vi "HDF5_Write_Tone_Record.vi"(0 "ToneRef":T5 {"Downshift_dset" format="%.0x"; "DeltaPhase_dset" format="%.0x"; "Phase_dset" format="%.0x"; "SNR_dset" format="%.0x"; "df_dset" format="%.0x"; "PeakLoc_dset" format="%.0x"; "MaxValue_dset" format="%.0x"; "TImeStamp_dset" format="%.0x"; "TimeString_dset" format="%.0x"}, 5 "TargetToneData":T1={"Cal"={"Shift_"=-24999462.633451957, "Peak_ToFPGA"=-24999462.633451957, "MaxValue"=0.0, "MaxIndex"=0, "Tone"={"PkLocTrak"=0.0, "PkLocDisp"=0.0, "df_"=0.0, "ZoomPwr"=[], "Phase"=0.0, "PhaseOld"=0.0, "AboveThresh?"=FALSE, "MaxI"=0.0, "MaxQ"=0.0, "median"=0.0, "ISpect"=[], "QSpect"=[], "DeltaPhase"=0.0}, "TimeDomainI"=array[12500 elements], "TimeDomainQ"=[], "PwrSpectrum"=array[12500 elements], "RunningAvgFreq"=0.0, "ISpectPos"=[], "ISpectNeg"=[], "QSpectPos"=[], "QSpectNeg"=[], "10Hz_PwrSpectr"=[], "SNR"=0.0, "AliasWarn"=FALSE, "10Hz_Peak"=[], "ISpect+-"=[], "QSpect+-"=[], "TimeStamp"=timestamp(0 s since 1904-01-01), "I_Index"=array[12500 elements], "Q_Index"=array[12500 elements], "10MHz"=FALSE}, "Beac"={"Shift_"=-24999462.633451957, "Peak_ToFPGA"=-24999462.633451957, "MaxValue"=0.0, "MaxIndex"=0, "Tone"={"PkLocTrak"=0.0, "PkLocDisp"=0.0, "df_"=0.0, "ZoomPwr"=[], "Phase"=0.0, "PhaseOld"=0.0, "AboveThresh?"=FALSE, "MaxI"=0.0, "MaxQ"=0.0, "median"=0.0, "ISpect"=[], "QSpect"=[], "DeltaPhase"=0.0}, "TimeDomainI"=array[12500 elements], "TimeDomainQ"=[], "PwrSpectrum"=array[12500 elements], "RunningAvgFreq"=0.0, "ISpectPos"=[], "ISpectNeg"=[], "QSpectPos"=[], "QSpectNeg"=[], "10Hz_PwrSpectr"=[], "SNR"=0.0, "AliasWarn"=FALSE, "10Hz_Peak"=[], "ISpect+-"=[], "QSpect+-"=[], "TimeStamp"=timestamp(0 s since 1904-01-01), "I_Index"=array[12500 elements], "Q_Index"=array[12500 elements], "10MHz"=FALSE}, "Time"=[], "Saturat"={"MeasMean0"=0.0, "MeasMean1"=0.0, "MeasMax"=0.0, "1_Max"=0.0, "4_Max"=0.0, "5_Max"=0.0, "6_Max"=0.0, "7_Max"=0.0}} {"Beac"."Tone"."median" format="%0.2f"; "Beac"."Tone"."MaxQ" format="%0.2f"; "Cal"."Tone"."median" format="%0.2f"; "Cal"."Tone"."MaxQ" format="%0.2f"}, 11 "error in":errorcluster) -> (15 "error out":errorcluster)   [LabVIEW 2018]
doc: "Write a single Tone<x> record with timestamp:\nTone1\n Beac - cluster\n BeacZoom - 1024 element Double array (waveform) \n Cal - cluster\n CalZoom - 1024 element Double array (waveform)"
uses:
  <vilib>/addons/h5labview2/dataset/H5D.lvlib
  <vilib>/addons/h5labview2/base/H5Equery.vi
  lib_path_mod_20200519.vi
  <vilib>/addons/h5labview2/dataset/H5Dwrite.llb/H5Dwrite.xnode
  <vilib>/addons/h5labview2/space/H5S.lvlib
  <vilib>/addons/h5labview2/base/hid_t_renamed.ctl
  HDF5_Tone_refs.ctl
  Controls/ToneInfoClust.ctl
  Controls/Clusts/ChannelToneData.ctl
  Controls/Clusts/TargetToneData.ctl
  Controls/Clusts/SaturationMonitor.ctl
  <vilib>/addons/h5labview2/base/hid_t.ctl
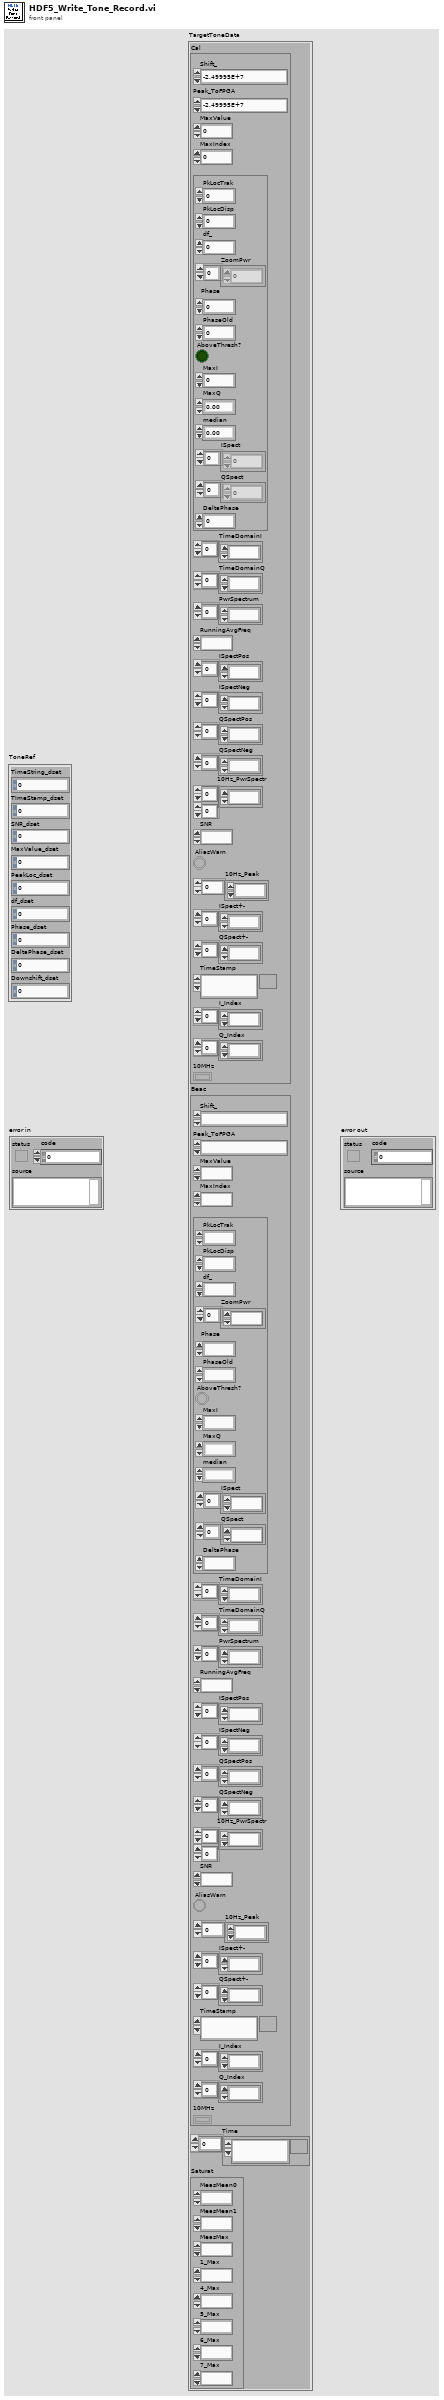
[diagram p1: front panel]
types:
  T1 = typedef "TargetToneData.ctl" = cluster{"Cal":T2, "Beac":T2, "Time":timestamp[], "Saturat":T4}
  T2 = typedef "ChannelToneData.ctl" = cluster{"Shift_":dbl, "Peak_ToFPGA":dbl, "MaxValue":dbl, "MaxIndex":i32, "Tone":T3, "TimeDomainI":ext[], "TimeDomainQ":ext[], "PwrSpectrum":dbl[], "RunningAvgFreq":dbl, "ISpectPos":dbl[], "ISpectNeg":dbl[], "QSpectPos":dbl[], "QSpectNeg":dbl[], "10Hz_PwrSpectr":dbl[][], "SNR":dbl, "AliasWarn":bool, "10Hz_Peak":dbl[], "ISpect+-":dbl[], "QSpect+-":dbl[], "TimeStamp":timestamp, "I_Index":ext[], "Q_Index":ext[], "10MHz":bool}
  T3 = typedef "ToneInfoClust.ctl" = cluster{"PkLocTrak":dbl, "PkLocDisp":dbl, "df_":dbl, "ZoomPwr":dbl[], "Phase":dbl, "PhaseOld":dbl, "AboveThresh?":bool, "MaxI":dbl, "MaxQ":dbl, "median":dbl, "ISpect":dbl[], "QSpect":dbl[], "DeltaPhase":dbl}
  T4 = typedef "SaturationMonitor.ctl" = cluster{"MeasMean0":dbl, "MeasMean1":dbl, "MeasMax":dbl, "1_Max":dbl, "4_Max":dbl, "5_Max":dbl, "6_Max":dbl, "7_Max":dbl}
  T5 = typedef "HDF5_Tone_refs.ctl" = cluster{"TimeString_dset":T6, "TImeStamp_dset":T6, "SNR_dset":T6, "MaxValue_dset":T6, "PeakLoc_dset":T6, "df_dset":T6, "Phase_dset":T6, "DeltaPhase_dset":T6, "Downshift_dset":T6}
  T6 = typedef "hid_t.ctl" = i32
  T7 = typedef "HDF5_ToneInfoClust.ctl" = cluster{"Timestring":string, "Timestamp":dbl, "MaxValue":dbl, "PeakLoc":dbl, "df":dbl}
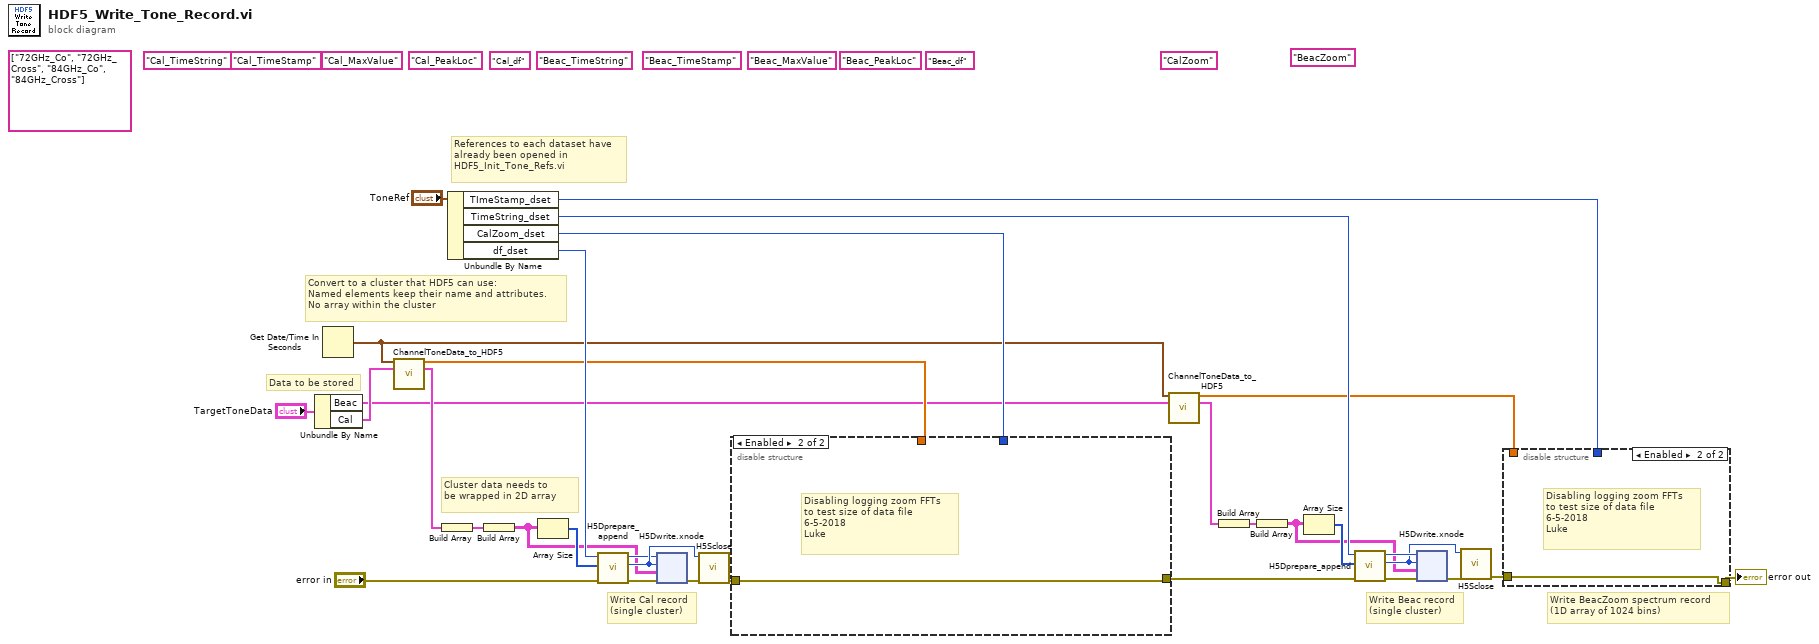
[diagram p0: block diagram]
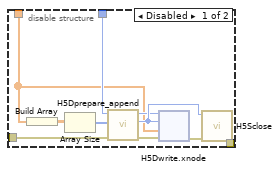
[diagram p2: hidden frame]
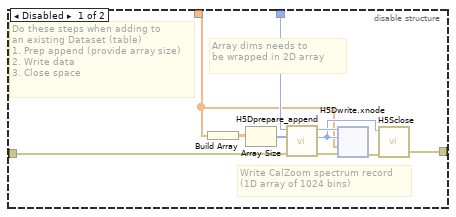
[diagram p3: hidden frame]
diagram:
  (unwired) "Beac_df" ("string")
  (unwired) "Beac_PeakLoc" ("string")
  (unwired) "Beac_MaxValue" ("string")
  w1 = "Beac_TimeStamp" ("string")
  w2 = "Beac_TimeString" ("string")
  (unwired) "Cal_df" ("string")
  (unwired) "Cal_PeakLoc" ("string")
  (unwired) "Cal_MaxValue" ("string")
  (unwired) "Cal_TimeStamp" ("string")
  (unwired) "BeacZoom" ("string")
  w3 = "CalZoom" ("string")
  (unwired) "Cal_TimeString" ("string")
  (unwired) string[] ["72GHz_Co", "72GHz_Cross", "84GHz_Co", "84GHz_Cross"]
  # "Convert to a cluster that HDF5 can use:\nNamed elements keep their name and attributes.\nNo array within the cluster"
  # "Cluster data needs to \nbe wrapped in 2D array"
  # "Data to be stored"
  # "References to each dataset have \nalready been opened in \nHDF5_Init_Tone_Refs.vi"
  # "Write BeacZoom spectrum record\n(1D array of 1024 bins)"
  # "Write Beac record\n(single cluster)"
  # "Write Cal record\n(single cluster)"
  n1 = Unbundle By Name("TargetToneData") -> ("Beac"=w10:T2, "Cal"=w14:T2)
  n2 = Get Date/Time In Seconds() -> (seconds since 1Jan1904=w9:timestamp)
  n3 = call "ChannelToneData_to_HDF5.vi"("Timestamp"=w9, "ChannelToneData"=w14) -> ("Zoom"=w11:dbl[], "HDF5_ToneData"=w13:T7)  [unwired: 12 in]
  n4 = Build Array(w13) -> (w22:T7[])
  n5 = Unbundle By Name("ToneRef") -> ("TImeStamp_dset"=w17:T6, "TimeString_dset"=w18:T6, "CalZoom_dset"=w19:T6, "df_dset"=w20:T6)
  n6 = Build Array(w22) -> (w12:T7[][])
  n7 = Array Size(array=w12) -> (size(s)=w16:i32[])
  n8 = call <vilib>:"H5Dprepare_append.vi"("error in (no error)"="error in", "append dims"=w16, "dset in"=w20) -> ("error out"=w35:errorcluster, "space out"=w33:T6, "dset out"=w32:T6)  [unwired: 5 in, 1 out]
  n9 = xnode "H5Dwrite.xnode"("error in (no error)"=w35, "data"=w12, "file space"=w33, "ref in"=w32) -> ("error out"=w34:errorcluster)  [unwired: 3 in, 2 out]
  n10 = call <vilib>:"H5Sclose.vi"("error in (no error)"=w34, "space in"=w33) -> ("error out"=w24:errorcluster)  [unwired: 9 in]
  n11 = disable-structure shown="Enabled" {
    disable-tunnel: [w41 w65] -> w25
    disable-tunnel: w24 -> [w40 w65]
    disable-tunnel: w19 -> [w39 _]
    disable-tunnel: w11 -> [w37 _]
    frame Disabled {
      # "Array dims needs to \nbe wrapped in 2D array"
      # "Do these steps when adding to \nan existing Dataset (table)\n1. Prep append (provide array size)\n2. Write data\n3. Close space"
      # "Write CalZoom spectrum record\n(1D array of 1024 bins)"
      n12 = Build Array(w37) -> (w38:dbl[][])
      n13 = Array Size(array=w38) -> (size(s)=w36:i32[])
      n14 = call <vilib>:"H5Dprepare_append.vi"("error in (no error)"=w40, "append dims"=w36, "dset in"=w39) -> ("error out"=w43:errorcluster, "space out"=w44:T6, "dset out"=w45:T6)  [unwired: 5 in, 1 out]
      n15 = xnode "H5Dwrite.xnode"("error in (no error)"=w43, "data"=w37, "file space"=w44, "ref in"=w45) -> ("error out"=w42:errorcluster)  [unwired: 3 in, 2 out]
      n16 = call <vilib>:"H5Sclose.vi"("error in (no error)"=w42, "space in"=w44) -> ("error out"=w41:errorcluster)  [unwired: 9 in]
    }
    frame Enabled {
      # "Disabling logging zoom FFTs\nto test size of data file\n6-5-2018\nLuke"
    }
  }
  n17 = call "ChannelToneData_to_HDF5.vi"("Timestamp"=w9, "ChannelToneData"=w10) -> ("Zoom"=w4:dbl[], "HDF5_ToneData"=w7:T7)  [unwired: 12 in]
  n18 = Build Array(w7) -> (w8:T7[])
  n19 = Build Array(w8) -> (w5:T7[][])
  n20 = Array Size(array=w5) -> (size(s)=w6:i32[])
  n21 = call <vilib>:"H5Dprepare_append.vi"("error in (no error)"=w25, "append dims"=w6, "dset in"=w18) -> ("error out"=w28:errorcluster, "space out"=w30:T6, "dset out"=w31:T6)  [unwired: 5 in, 1 out]
  n22 = xnode "H5Dwrite.xnode"("error in (no error)"=w28, "data"=w5, "file space"=w30, "ref in"=w31) -> ("error out"=w29:errorcluster)  [unwired: 3 in, 2 out]
  n23 = call <vilib>:"H5Sclose.vi"("error in (no error)"=w29, "space in"=w30) -> ("error out"=w26:errorcluster)  [unwired: 9 in]
  n24 = disable-structure shown="Enabled" {
    disable-tunnel: [w71 w95] -> w27
    disable-tunnel: w26 -> [w70 w95]
    disable-tunnel: w17 -> [w69 _]
    disable-tunnel: w4 -> [w66 _]
    frame Disabled {
      n25 = Build Array(w66) -> (w68:dbl[][])
      n26 = Array Size(array=w68) -> (size(s)=w67:i32[])
      n27 = call <vilib>:"H5Dprepare_append.vi"("error in (no error)"=w70, "append dims"=w67, "dset in"=w69) -> ("error out"=w74:errorcluster, "space out"=w73:T6, "dset out"=w72:T6)  [unwired: 5 in, 1 out]
      n28 = xnode "H5Dwrite.xnode"("error in (no error)"=w74, "data"=w66, "file space"=w73, "ref in"=w72) -> ("error out"=w75:errorcluster)  [unwired: 3 in, 2 out]
      n29 = call <vilib>:"H5Sclose.vi"("error in (no error)"=w75, "space in"=w73) -> ("error out"=w71:errorcluster)  [unwired: 9 in]
    }
    frame Enabled {
      # "Disabling logging zoom FFTs\nto test size of data file\n6-5-2018\nLuke"
    }
  }
  "error out" <- w27
